vi "T9.vi"() -> ()   [LabVIEW 2020]
panel:
  out "SUMA":dbl
  in  "B":dbl
  in  "A":dbl
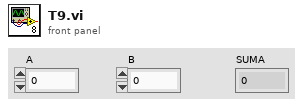
[diagram p1: front panel]
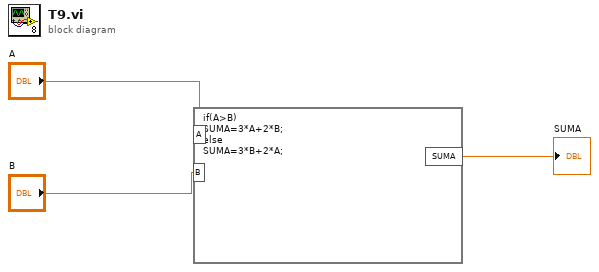
[diagram p0: block diagram]
diagram:
  n1 = formula code="if(A>B)\nSUMA=3*A+2*B;\nelse\nSUMA=3*B+2*A;"("A"="A", "B"="B") -> ("SUMA"=→"SUMA":dbl)
